vi "Define Parameter.vi"(8 "error in (no error)":errorcluster, 11 "Analyze Fluence in":refnum<class "Analyze Fluence.lvclass">) -> (0 "error out":errorcluster, 3 "Analyze Fluence out":refnum<class "Analyze Fluence.lvclass">)   [LabVIEW 2020, in "Analyze.lvlib" / "Analyze Fluence.lvclass"]
uses:
  Analyze Fluence.lvclass
  Analyze Parameter/Analyze Parameter Fluence/Analyze Parameter Fluence.lvclass
  C:/POLARIS Programme/POLARIS-AS-3-Cams/Submodules/HIJ Vision/Analyze/Analyze Parameter/Analyze Parameter Base/Analyze Parameter Base.lvclass
  Analyze Parameter/Analyze Parameter Energy/Analyze Parameter Energy.lvclass
  Analyze BaseClass/Analyze BaseClass/Analyze BaseClass.lvclass
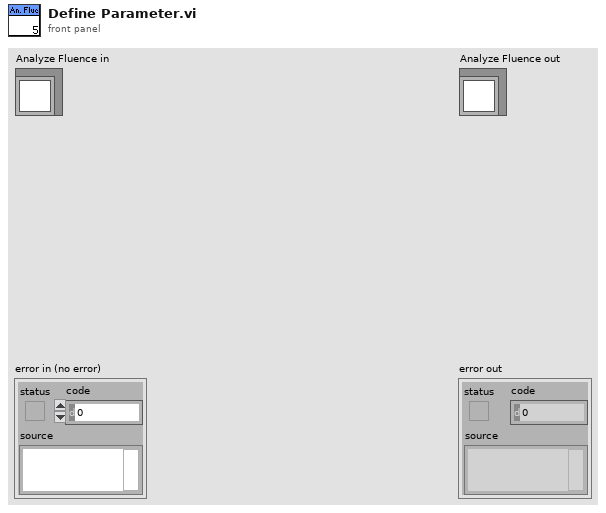
[diagram p1: front panel]
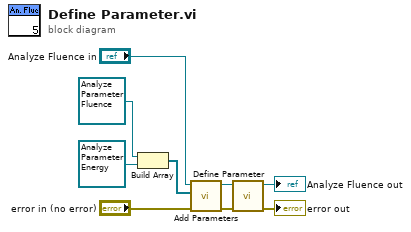
[diagram p0: block diagram]
diagram:
  n1 = Build Array(refnum<class "Analyze Parameter Fluence.lvclass"> refnum ("Parameter"), refnum<class "Analyze Parameter Energy.lvclass"> refnum ("Energy")) -> (w5:refnum<class "Analyze Parameter Base.lvclass">[])
  n2 = call-dynamic "Add Parameters.vi"("error in (no error)"="error in (no error)", "Parameters"=w5, "Analyze BaseClass in"="Analyze Fluence in") -> ("error out"=w1:errorcluster, "Analyze BaseClass out"=w2:refnum<class "Analyze Fluence.lvclass">)  [unwired: 7 in]
  n3 = call-parent "Define Parameter.vi"("error in (no error)"=w1, "Analyze BaseClass in"=w2) -> ("error out"=→"error out":errorcluster, "Analyze BaseClass out"=→"Analyze Fluence out":refnum<class "Analyze Fluence.lvclass">)  [unwired: 8 in]
